vi "mergeVariablePropertyNode.vi"   [LabVIEW 2020]
doc: "Gets (reads) and/or sets (writes) properties of a reference. This node operates the same way as a standard Property Node. However, this node is pre-configured for Variable references."
uses:
  <resource>/objmgr/ni.var.rc
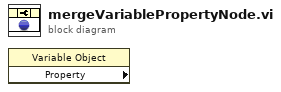
[diagram p0: block diagram]
diagram:
  n1 = property class="Variable Object" props=[]() -> ()  [unwired: 2 in, 3 out]
